vi "Write I2C.vi"(5 "Address":u8, 6 "NoStop (F)":bool, 7 "Bus":u8, 8 "error in (no error)":errorcluster, 10 "Data":string, 11 "VISA resource name in":refnum<visa-resource-name>) -> (0 "error out":errorcluster, 3 "VISA resource name":refnum<visa-resource-name>)   [LabVIEW 2023, in "CTI-Visa.lvlib"]
uses:
  CTI-Visa.lvlib
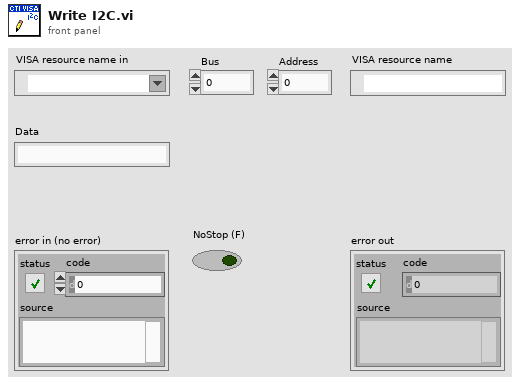
[diagram p1: front panel]
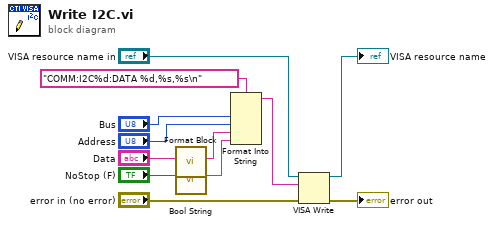
[diagram p0: block diagram]
diagram:
  n1 = call "Format Block.vi"("Data Block"="Data") -> ("Formatted Block"=w9:string)  [unwired: 10 in]
  n2 = call "Bool String.vi"("Bool"="NoStop (F)") -> ("String"=w8:string)  [unwired: 10 in]
  n3 = Format Into String(format string="COMM:I2C%d:DATA %d,%s,%s\n", "Bus", "Address", w9, w8) -> (resulting string=w5:string)  [unwired: 2 in, 1 out]
  n4 = VISA Write(VISA resource name="VISA resource name in", write buffer=w5, error in (no error)="error in (no error)") -> (VISA resource name out=→"VISA resource name":refnum<visa-resource-name>, error out=→"error out":errorcluster)  [unwired: 1 out]
